vi "Untitled 2.vi"() -> ()   [LabVIEW 2016]
panel:
  in  "Boolean":bool
  out "Numeric":dbl
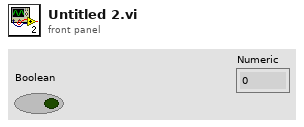
[diagram p1: front panel]
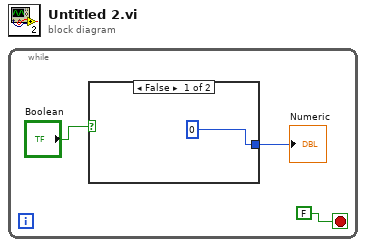
[diagram p0: block diagram]
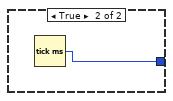
[diagram p2: hidden frame]
diagram:
  n1 = while {
    stop <- FALSE stop-if-true
    n2 = case shown="False" "Boolean" {
      tunnel: [0 w5] -> w3
      frame False {
      }
      frame True {
        n3 = Tick Count (ms)() -> (millisecond timer value=w5:u32)
      }
    }
    "Numeric" <- w3
  }
